vi "Write Record Data.vi"(8 "Error In (no error)":errorcluster, 10 "Record":variant, 11 "Expenses Tracker Transaction In":refnum<class "Expenses Tracker Transaction.lvclass">) -> (0 "Error Out":errorcluster, 3 "Expenses Tracker Transaction Out":refnum<class "Expenses Tracker Transaction.lvclass">)   [LabVIEW 2023, in "Expenses Tracker Transaction.lvclass"]
uses:
  Expenses Tracker Transaction.lvclass
  Ctrls/Transaction.ctl
  Expenses Tracker Transaction.lvclass/Expenses Tracker Transaction.ctl
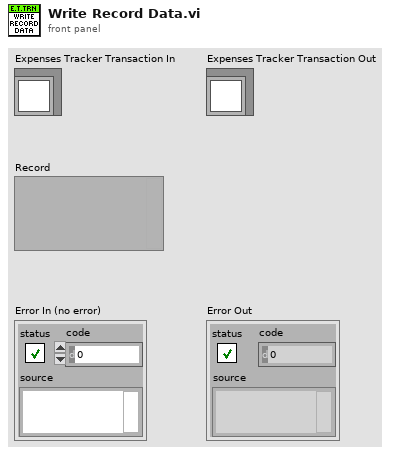
[diagram p1: front panel]
types:
  T1 = typedef "Expenses Tracker Transaction.lvclass/Transaction.ctl" = cluster{"ID":u32, "Name":string, "Is_income":bool, "Value":dbl, "Amount":dbl, "Total":dbl, "Date_of_entry":timestamp, "Date_of_occurence":timestamp, "Last_update":timestamp, "Category":u32, "Subcategory":u32, "Cycle":u32, "Description":string}
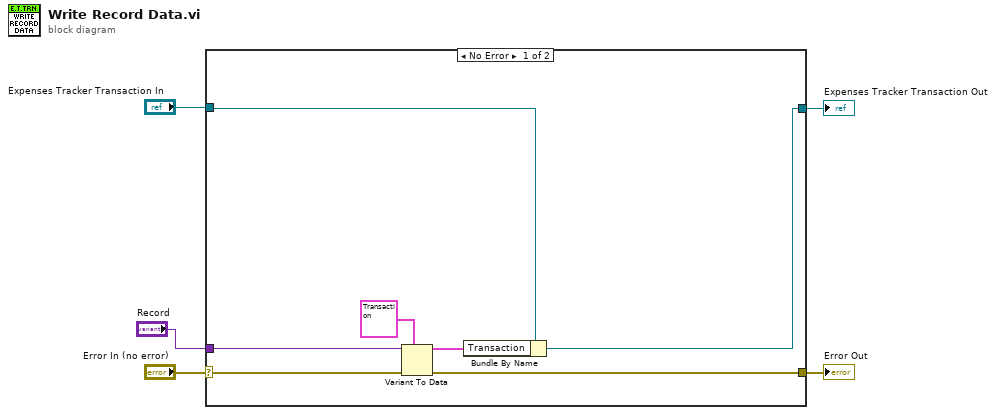
[diagram p0: block diagram]
diagram:
  n1 = case shown="No Error" "Error In (no error)" {
    selector: "Error In (no error)" -> [w11 w14]
    tunnel: [w9 w14] -> w5
    tunnel: [w7 w13] -> w2
    tunnel: "Expenses Tracker Transaction In" -> [w8 w13]
    tunnel: "Record" -> [w12 _]
    frame No Error {
      n2 = Variant To Data(error in=w11, type=T1 {"ID"=0, "Name"="", "Is_income"=FALSE, "Value"=0.0, "Amount"=0.0, "Total"=0.0, "Date_of_entry"=timestamp(0 s since 1904-01-01), "Date_of_occurence"=timestamp(0 s since 1904-01-01), "Last_update"=timestamp(0 s since 1904-01-01), "Category"=0, "Subcategory"=0, "Cycle"=0, "Description"=""} ("Transaction"), Variant=w12) -> (data=w6:T1, error out=w9:errorcluster)
      n3 = Bundle By Name(cluster=w8, "Transaction"=w6) -> (w7:refnum<class "Expenses Tracker Transaction.lvclass">)
    }
    frame Error {
    }
  }
  "Error Out" <- w5
  "Expenses Tracker Transaction Out" <- w2
